vi "Run All Tests.vi"   [LabVIEW 2021]
uses:
  <vilib>/addons/_JKI Toolkits/Caraya/run-tests/Run Test (Scalar Path).vi
  <vilib>/addons/_JKI Toolkits/Caraya/Caraya.lvlib
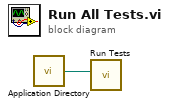
[diagram p0: block diagram]
diagram:
  n1 = call <vilib>:"Application Directory.vi"() -> ("Application Directory"=w1:path)
  n2 = call-poly <vilib>:"Run Tests.vi"("Test Path"=w1) -> ()  [unwired: 9 in, 2 out]
